vi "Destroy All Message Queues.vi"(8 "error in (no error)":errorcluster, 11 "Message Queues":T1) -> (0 "error out":errorcluster)   [LabVIEW 2014, in "Message Queue.lvlib"]
doc: "This VI creates and initializes all the message queues for your application. If your application requires more than one message queue, right-click the \"Message Queues\" constant above and select Open Type Def. Add the new Message Queue(s) to the type definition, then initialize them in this VI."
uses:
  Message Queue.lvlib
  All Message Queues.ctl
  Message Cluster.ctl
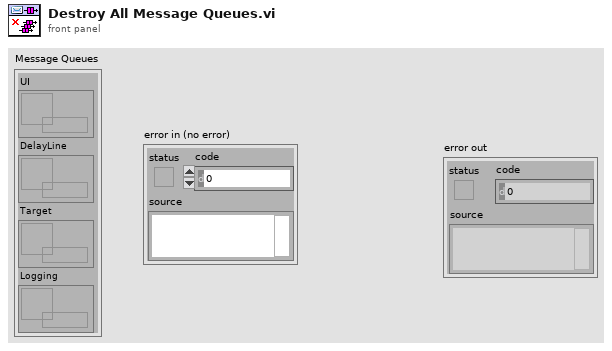
[diagram p1: front panel]
types:
  T1 = typedef "Message Queue.lvlib/All Message Queues.ctl" = cluster{"UI":refnum<queue>, "DelayLine":refnum<queue>, "Target":refnum<queue>, "Logging":refnum<queue>}
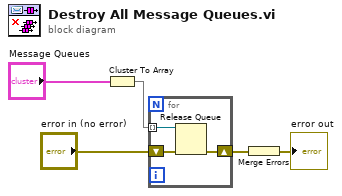
[diagram p0: block diagram]
diagram:
  n1 = Cluster To Array(cluster="Message Queues") -> (array=w1:refnum<queue>[])
  n2 = for {
    shift-right: [w7] -> w3
    shift-left: "error in (no error)" -> [w8]
    tunnel: w1 -> [w6] mode=indexing
    n3 = Release Queue(queue=w6, error in (no error)=w8) -> (error out=w7:errorcluster)  [unwired: 1 in, 2 out]
  }
  n4 = Merge Errors(w3) -> (→"error out":errorcluster)
